vi "Return Data Packet.vi"(7 "Connection ID":string, 8 "error in (no error)":errorcluster, 9 "Packet Data":variant, 10 "Packet Header":string, 11 "IPacketReturn in":refnum<class "IPacket Return.lvclass">) -> (0 "error out":errorcluster)   [LabVIEW 2019, in "Network Messenger.lvlib" / "IPacket Return.lvclass"]
uses:
  <vilib>/gpm_packages/@cs/Network-interface/Source/Network Messenger/IPacket Return/IPacket Return.lvclass
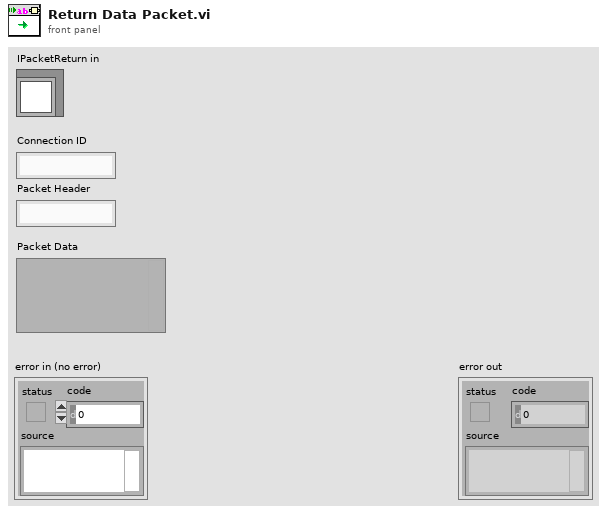
[diagram p1: front panel]
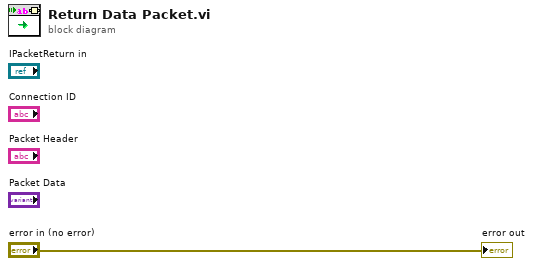
[diagram p0: block diagram]
diagram:
  "error out" <- "error in (no error)"
